vi "TaskNameFromChannels.vi"(5 "I/O Channels":refnum<k21>[](array[refnum])) -> (2 "Task Name":string)   [LabVIEW 2013]
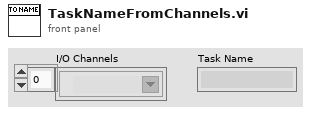
[diagram p1: front panel]
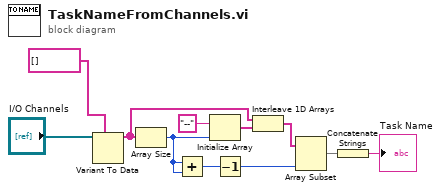
[diagram p0: block diagram]
diagram:
  n1 = Variant To Data(type=string[] [] ("names in"), Variant="I/O Channels") -> (data=w4:string[])  [unwired: 1 in, 1 out]
  n2 = Array Size(array=w4) -> (size(s)=w9:i32)
  n3 = Add(x=w9, y=w9) -> (x+y=w10:i32)
  n4 = Initialize Array("--", w9) -> (w5:string[])
  n5 = Decrement(x=w10) -> (x-1=w11:i32)
  n6 = Interleave 1D Arrays(w4, w5) -> (w7:string[])
  n7 = Array Subset(array=w7, length=w11) -> (w8:string[])  [unwired: 1 in]
  n8 = Concatenate Strings(w8) -> (→"Task Name":string)
